vi "GVSView Global.vi"() -> ()   [LabVIEW 2013]
uses:
  <vilib>/Utility/miscctls.llb/LVRectTypeDef.ctl
panel:
  in  "cCurverOutDataList":T1(array[cluster])
  in  "sActiveView":string
  in  "nDBGTempleteCount":i32
  in  "DBGLoadSplitterList":T2(array[cluster])
  in  "DBGSaveSplitterList":T2(array[cluster])
  out "ResultInCurLibrary":T3={"bResult"=TRUE, "SData_Out"="", "pVIRef_Out"=refnum, "pVIRefList_Out"=[]}
  in  "ViewCommand":T4
  out "VIRefCommandQueue":refnum<vi>
  in  "ViewCommandList":T5(array[cluster])
  out "DestVIRef":refnum<vi>
  in  "SourSPRef":refnum<vi>
  in  "SourSPVRef":refnum<vi>
  in  "SourSPHRef":refnum<vi>
  in  "SetGraphDataList":cluster{"sAction":string, "sData":string}[](array[cluster])
  in  "cSplitterList":T2(array[cluster])
  in  "cSplitter":T6
  out "sUseView":string
  in  "cBootDATAVIEW":T7
  out "sDockingType":string
  in  "nDockSourIDF":i32
  in  "nDockDestIDF":i32
  in  "DockingBounds":T8
  in  "DockViewBounds":T8
  in  "DockDestBounds":T8
  in  "VritualBounds":T8
  out "sDefaultGraph":string="XY"
  in  "cViewList":T9
  in  "cBootVIEW":T7
  in  "cMSG":T10
  in  "cCurverOutData":T11
  out "VIRefOuting":refnum<vi>
  in  "cVIEWFrame":T12
  in  "cTab":T13
  in  "cWiin":T14
  in  "cFrame":T15
  in  "cView":T16
  in  "pathViewLog":path
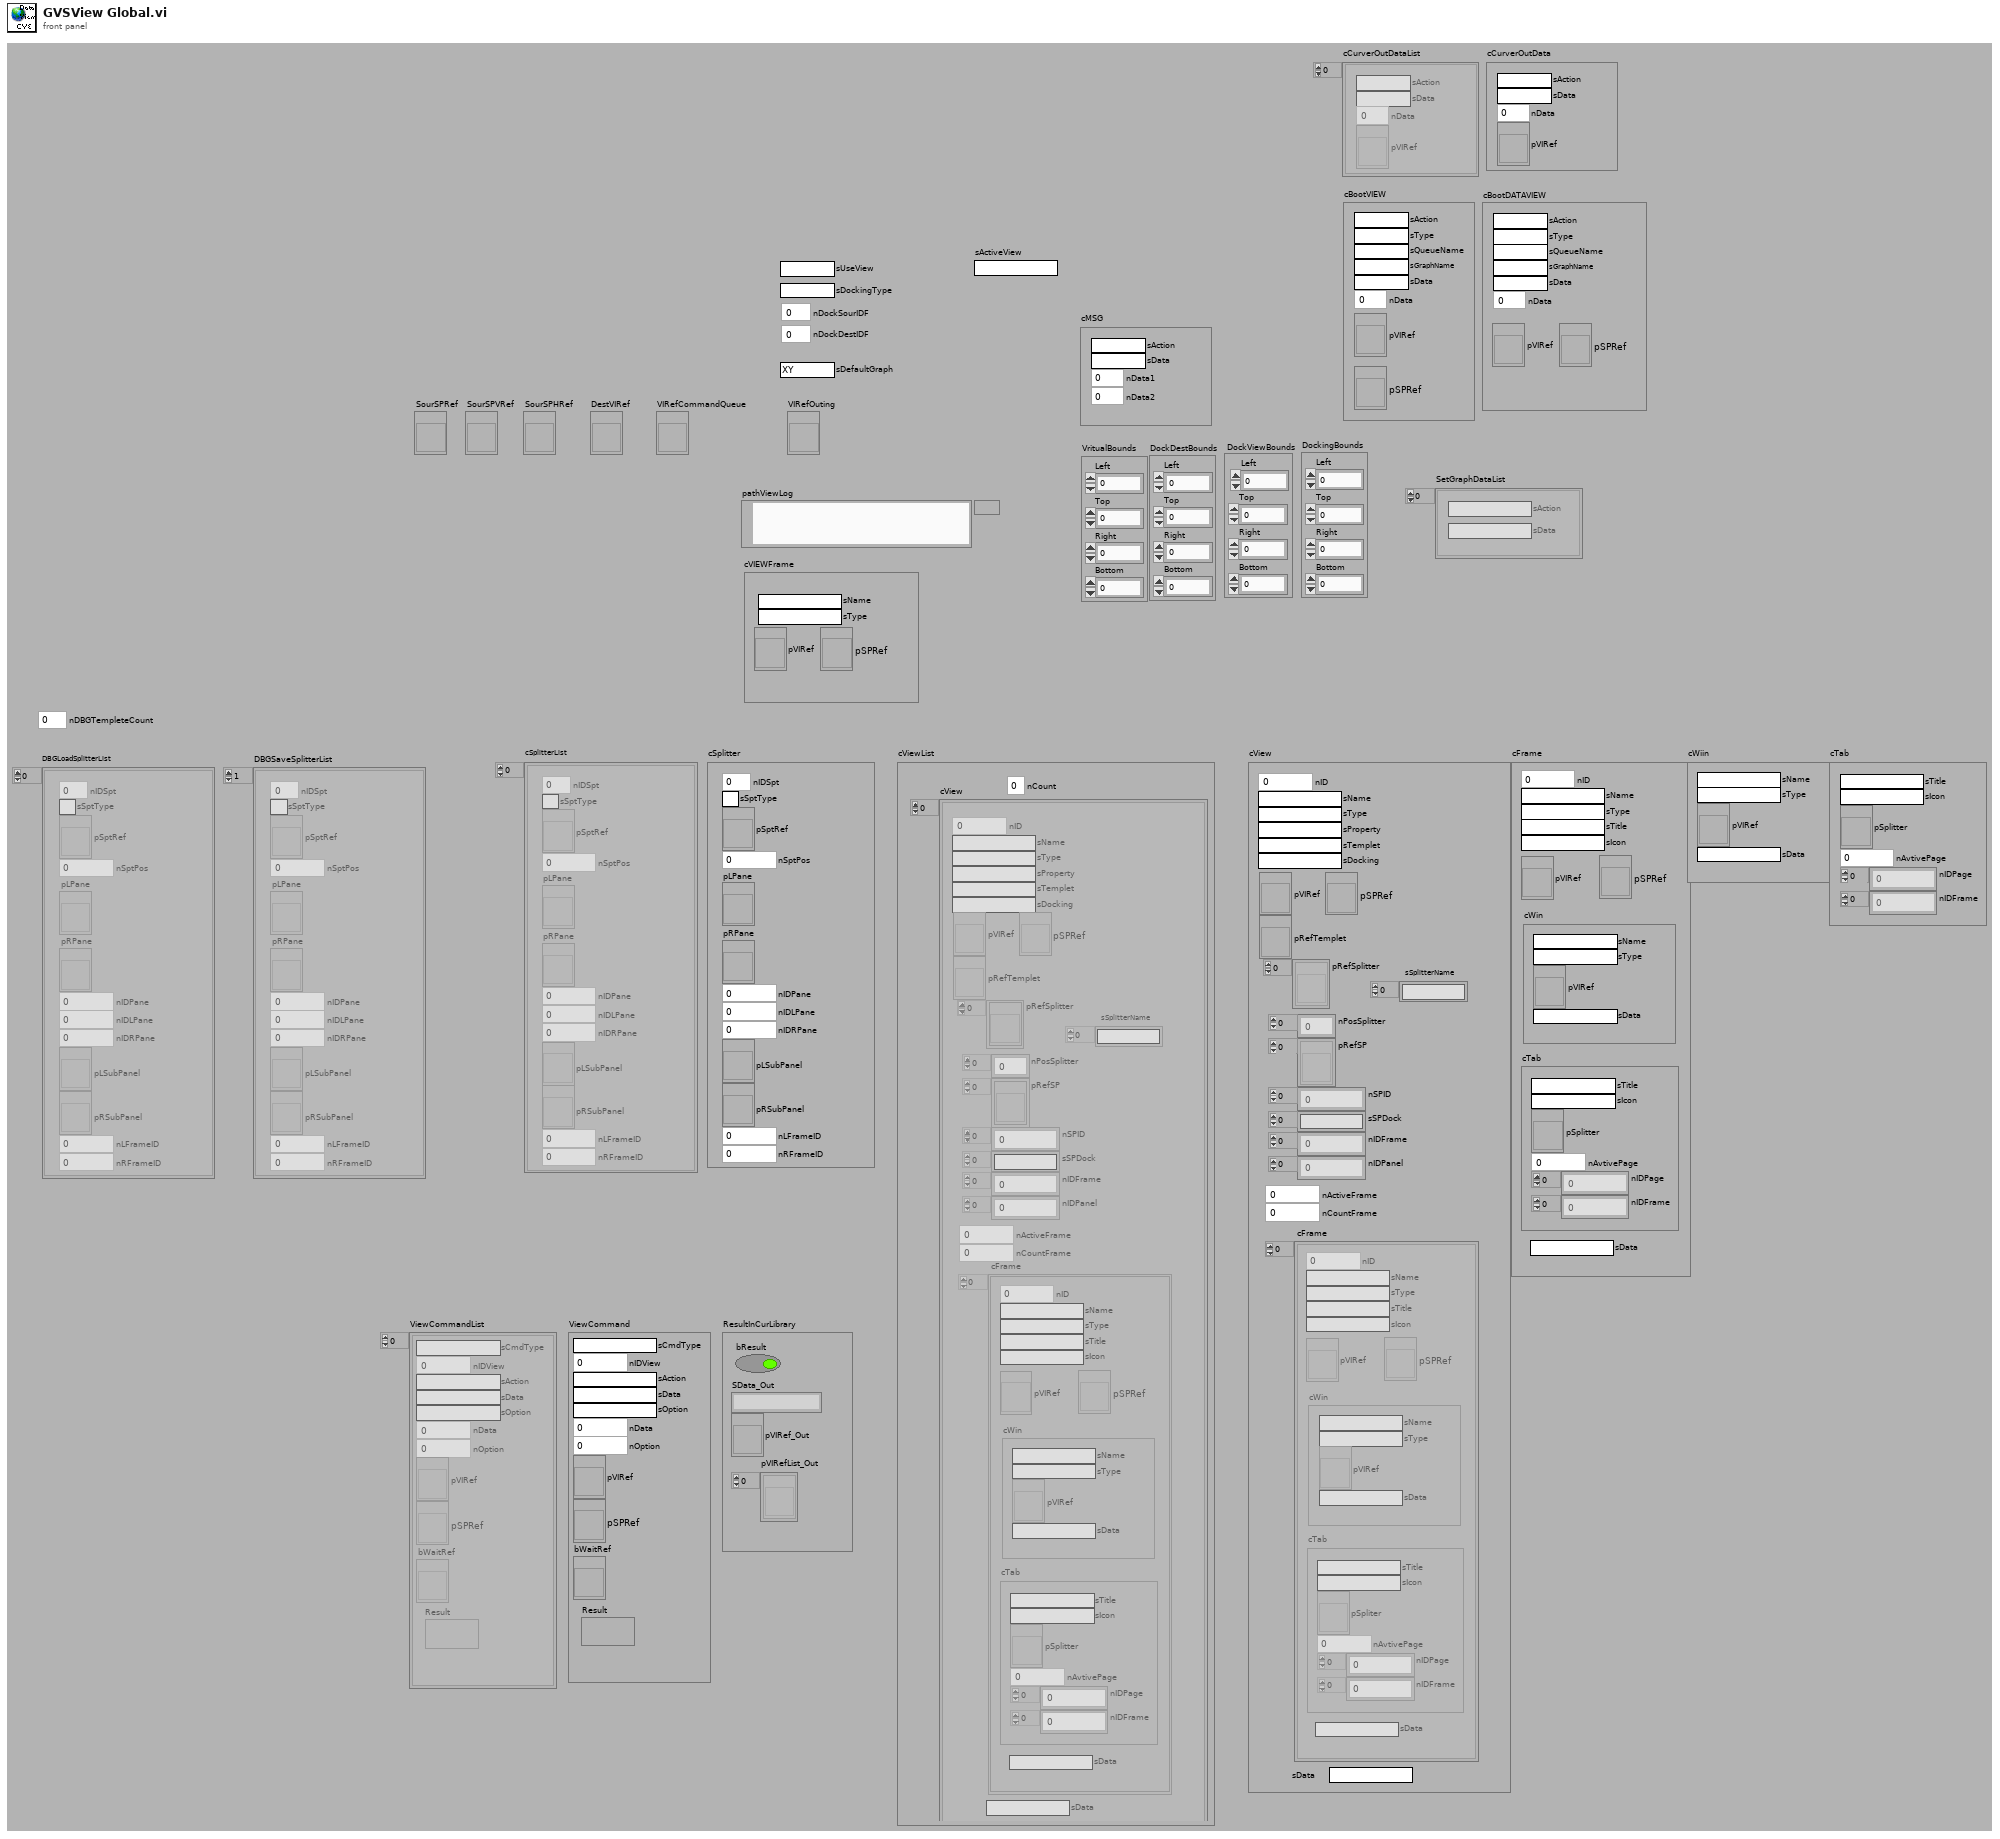
[diagram p1: front panel]
types:
  T1 = cluster{"sAction":string, "sData":string, "nData":i32, "pVIRef":refnum<vi>}[]
  T2 = cluster{"nIDSpt":i32, "sSptType":string, "pSptRef":refnum<vi>, "nSptPos":i32, "pLPane":refnum<vi>, "pRPane":refnum<vi>, "nIDPane":i32, "nIDLPane":i32, "nIDRPane":i32, "pLSubPanel":refnum<vi>, "pRSubPanel":refnum<vi>, "nLFrameID":i32, "nRFrameID":i32}[]
  T3 = cluster{"bResult":bool, "SData_Out":string, "pVIRef_Out":refnum<vi>, "pVIRefList_Out":refnum<vi>[]}
  T4 = cluster{"sCmdType":string, "nIDView":i32, "sAction":string, "sData":string, "sOption":string, "nData":i32, "nOption":i32, "pVIRef":refnum<vi>, "pSPRef":refnum<vi>, "bWaitRef":refnum<vi>, "Result":variant}
  T5 = cluster{"sCmdType":string, "nIDView":i32, "sAction":string, "sData":string, "sOption":string, "nData":i32, "nOption":i32, "pVIRef":refnum<vi>, "pSPRef":refnum<vi>, "bWaitRef":refnum<vi>, "Result":variant}[]
  T6 = cluster{"nIDSpt":i32, "sSptType":string, "pSptRef":refnum<vi>, "nSptPos":i32, "pLPane":refnum<vi>, "pRPane":refnum<vi>, "nIDPane":i32, "nIDLPane":i32, "nIDRPane":i32, "pLSubPanel":refnum<vi>, "pRSubPanel":refnum<vi>, "nLFrameID":i32, "nRFrameID":i32}
  T7 = cluster{"sAction":string, "sType":string, "sQueueName":string, "sGraphName":string, "sData":string, "nData":i32, "pVIRef":refnum<vi>, "pSPRef":refnum<vi>}
  T8 = typedef "LVRectTypeDef.ctl" = cluster{"Left":i16, "Top":i16, "Right":i16, "Bottom":i16}
  T9 = cluster{"nCount":i32, "cView":cluster{"nID":i32, "sName":string, "sType":string, "sProperty":string, "sTemplet":string, "sDocking":string, "pVIRef":refnum<vi>, "pSPRef":refnum<vi>, "pRefTemplet":refnum<vi>, "pRefSplitter":refnum<vi>[], "nPosSplitter":i32[], "pRefSP":refnum<vi>[], "nSPID":i32[], "sSPDock":string[], "nIDFrame":i32[], "nIDPanel":i32[], "nActiveFrame":i32, "nCountFrame":i32, "cFrame":cluster{"nID":i32, "sName":string, "sType":string, "sTitle":string, "sIcon":string, "pVIRef":refnum<vi>, "pSPRef":refnum<vi>, "cWin":cluster{"sName":string, "sType":string, "pVIRef":refnum<vi>, "sData":string}, "cTab":cluster{"sTitle":string, "sIcon":string, "pSplitter":refnum<vi>, "nAvtivePage":i32, "nIDPage":i32[], "nIDFrame":i32[]}, "sData":string}[], "sData":string, "sSplitterName":string[]}[]}
  T10 = cluster{"sAction":string, "sData":string, "nData1":i32, "nData2":i32}
  T11 = cluster{"sAction":string, "sData":string, "nData":i32, "pVIRef":refnum<vi>}
  T12 = cluster{"sName":string, "sType":string, "pVIRef":refnum<vi>, "pSPRef":refnum<vi>}
  T13 = cluster{"sTitle":string, "sIcon":string, "pSplitter":refnum<vi>, "nAvtivePage":i32, "nIDPage":i32[], "nIDFrame":i32[]}
  T14 = cluster{"sName":string, "sType":string, "pVIRef":refnum<vi>, "sData":string}
  T15 = cluster{"nID":i32, "sName":string, "sType":string, "sTitle":string, "sIcon":string, "pVIRef":refnum<vi>, "pSPRef":refnum<vi>, "cWin":cluster{"sName":string, "sType":string, "pVIRef":refnum<vi>, "sData":string}, "cTab":cluster{"sTitle":string, "sIcon":string, "pSplitter":refnum<vi>, "nAvtivePage":i32, "nIDPage":i32[], "nIDFrame":i32[]}, "sData":string}
  T16 = cluster{"nID":i32, "sName":string, "sType":string, "sProperty":string, "sTemplet":string, "sDocking":string, "pVIRef":refnum<vi>, "pSPRef":refnum<vi>, "pRefTemplet":refnum<vi>, "pRefSplitter":refnum<vi>[], "nPosSplitter":i32[], "pRefSP":refnum<vi>[], "nSPID":i32[], "sSPDock":string[], "nIDFrame":i32[], "nIDPanel":i32[], "nActiveFrame":i32, "nCountFrame":i32, "cFrame":cluster{"nID":i32, "sName":string, "sType":string, "sTitle":string, "sIcon":string, "pVIRef":refnum<vi>, "pSPRef":refnum<vi>, "cWin":cluster{"sName":string, "sType":string, "pVIRef":refnum<vi>, "sData":string}, "cTab":cluster{"sTitle":string, "sIcon":string, "pSpliter":refnum<vi>, "nAvtivePage":i32, "nIDPage":i32[], "nIDFrame":i32[]}, "sData":string}[], "sData":string, "sSplitterName":string[]}
diagram:
